vi "全局 1.vi"() -> ()   [LabVIEW 2022 SP3]
panel:
  out "ENC滤波长度":dbl
  out "ENC滤波":dbl
  out "ENC滤波辅助":dbl[](array[numeric])
  out "ENC初始值":u16
  out "获得初始值":bool
  out "是否匀速转动":bool
  out "启动":bool
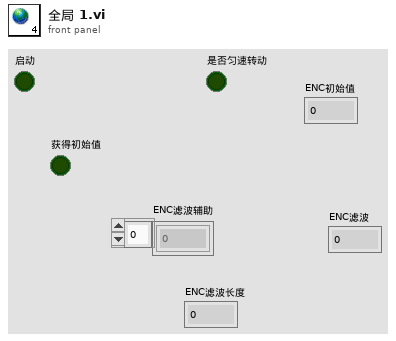
[diagram p1: front panel]
diagram:
